vi "ApplyStamp.vi"() -> ()   [LabVIEW 2017]
uses:
  Gantry/Shared Components/Gantry Class/Type Definitions/Virtual Modes.ctl
  Gantry/Shared Components/Gantry Class/Gantry.lvclass
  Gantry/Shared Components/FlexWorktable/FlexWorktable.lvclass
  Gantry/Shared Components/Vec3d Class/Vec3d.lvclass
panel:
  out "error out":errorcluster
  in  "Config Folder":path=path "C:/Users/husker/Desktop/gantry/Config"
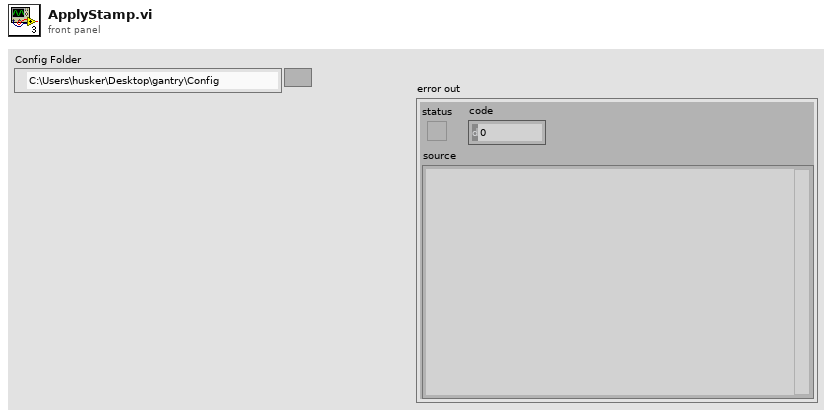
[diagram p1: front panel]
types:
  T1 = typedef "Virtual Modes.ctl" = enum16{"Nonvirtual", "Virtual"}
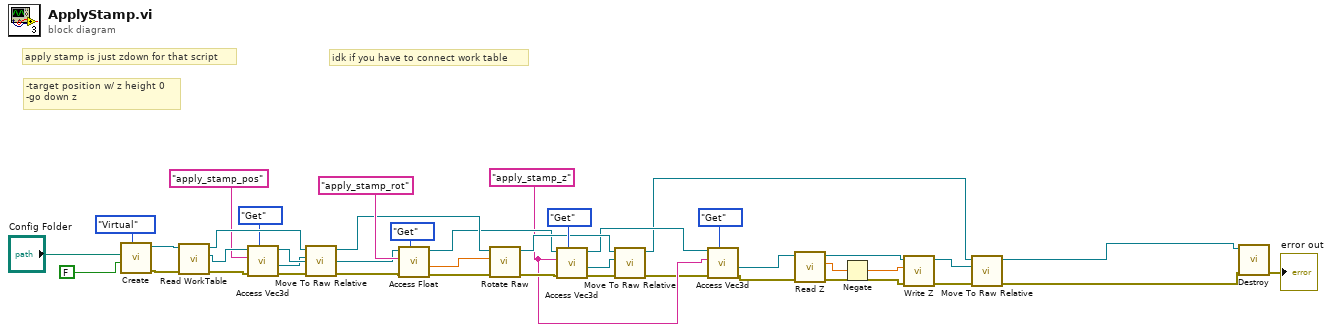
[diagram p0: block diagram]
diagram:
  w13 = "apply_stamp_z" ("Key")
  # "idk if you have to connect work table"
  # "-target position w/ z height 0\n-go down z"
  # "apply stamp is just zdown for that script"
  n1 = call "Create.vi"("Virtual Mode"=Virtual_Modes."Virtual", "HOME?"=FALSE, "Config Folder"="Config Folder") -> ("error out"=w36:errorcluster, "Gantry out"=w37:refnum<class "Gantry.lvclass">)  [unwired: 6 in, 1 out]
  n2 = call-dynamic "Read WorkTable.vi"("error in"=w36, "Gantry Class in"=w37) -> ("error out"=w29:errorcluster, "Worktable"=w31:refnum<class "FlexWorktable.lvclass">, "Gantry Class out"=w30:refnum<class "Gantry.lvclass">)  [unwired: 7 in]
  n3 = call-dynamic "Access Vec3d.vi"("Get/Set"=enum16{"Get", "Set"}."Get", "error in (no error)"=w29, "Key"="apply_stamp_pos", "FlexWorktable in"=w31) -> ("error out"=w28:errorcluster, "Value out"=w17:refnum<class "Vec3d.lvclass">, "FlexWorktable out"=w19:refnum<class "FlexWorktable.lvclass">)  [unwired: 5 in]
  n4 = call-dynamic "Move To Raw Relative.vi"("error in"=w28, "Delta"=w17, "Gantry in"=w30) -> ("error out"=w26:errorcluster, "Gantry out"=w25:refnum<class "Gantry.lvclass">)  [unwired: 7 in]
  n5 = call-dynamic "Access Float.vi"("Get/Set"=enum16{"Get", "Set"}."Get", "error in (no error)"=w26, "Key"="apply_stamp_rot", "FlexWorktable in"=w19) -> ("error out"=w35:errorcluster, "Value out"=w33:dbl, "FlexWorktable out"=w18:refnum<class "FlexWorktable.lvclass">)  [unwired: 5 in]
  n6 = call-dynamic "Rotate Raw.vi"("error in"=w35, "position(deg)"=w33, "Gantry in"=w25) -> ("error out"=w20:errorcluster, "Gantry out"=w21:refnum<class "Gantry.lvclass">)  [unwired: 7 in]
  n7 = call-dynamic "Access Vec3d.vi"("Get/Set"=enum16{"Get", "Set"}."Get", "error in (no error)"=w20, "Key"=w13, "FlexWorktable in"=w18) -> ("error out"=w23:errorcluster, "Value out"=w16:refnum<class "Vec3d.lvclass">, "FlexWorktable out"=w14:refnum<class "FlexWorktable.lvclass">)  [unwired: 5 in]
  n8 = call-dynamic "Move To Raw Relative.vi"("error in"=w23, "Delta"=w16, "Gantry in"=w21) -> ("error out"=w12:errorcluster, "Gantry out"=w3:refnum<class "Gantry.lvclass">)  [unwired: 7 in]
  n9 = call-dynamic "Access Vec3d.vi"("Get/Set"=enum16{"Get", "Set"}."Get", "error in (no error)"=w12, "Key"=w13, "FlexWorktable in"=w14) -> ("error out"=w10:errorcluster, "Value out"=w11:refnum<class "Vec3d.lvclass">)  [unwired: 5 in, 1 out]
  n10 = call-dynamic "Read Z.vi"("error in (no error)"=w10, "Vec3d Class in"=w11) -> ("error out"=w6:errorcluster, "Z"=w9:dbl, "Vec3d Class out"=w7:refnum<class "Vec3d.lvclass">)  [unwired: 7 in]
  n11 = Negate(x=w9) -> (-x=w8:dbl)
  n12 = call-dynamic "Write Z.vi"("error in (no error)"=w6, "Z"=w8, "Vec3d Class in"=w7) -> ("error out"=w4:errorcluster, "Vec3d Class out"=w5:refnum<class "Vec3d.lvclass">)  [unwired: 7 in]
  n13 = call-dynamic "Move To Raw Relative.vi"("error in"=w4, "Delta"=w5, "Gantry in"=w3) -> ("error out"=w1:errorcluster, "Gantry out"=w2:refnum<class "Gantry.lvclass">)  [unwired: 7 in]
  n14 = call "Destroy.vi"("error in"=w1, "Gantry Class in"=w2) -> ("error out"=→"error out":errorcluster)  [unwired: 9 in]
